vi "StartSession.vi"(8 "error in (no error)":errorcluster, 11 "TrialBasedExperiment in":refnum<class "MatlabExperiment.lvclass">) -> (0 "error out":errorcluster, 3 "TrialBasedExperiment out":refnum<class "MatlabExperiment.lvclass">)   [LabVIEW 2014, in "AcquisitionCoreObjects.lvlib" / "MatlabExperiment.lvclass"]
uses:
  MatlabExperiment.lvclass
  TrialBasedExperimentObject/TrialBasedExperiment.lvclass
  Matlab API/Matlab API.lvlib
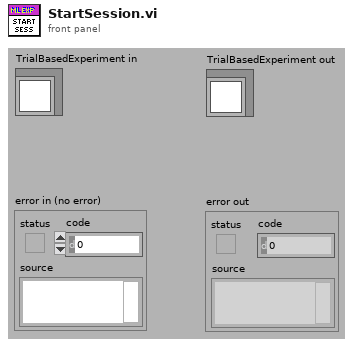
[diagram p1: front panel]
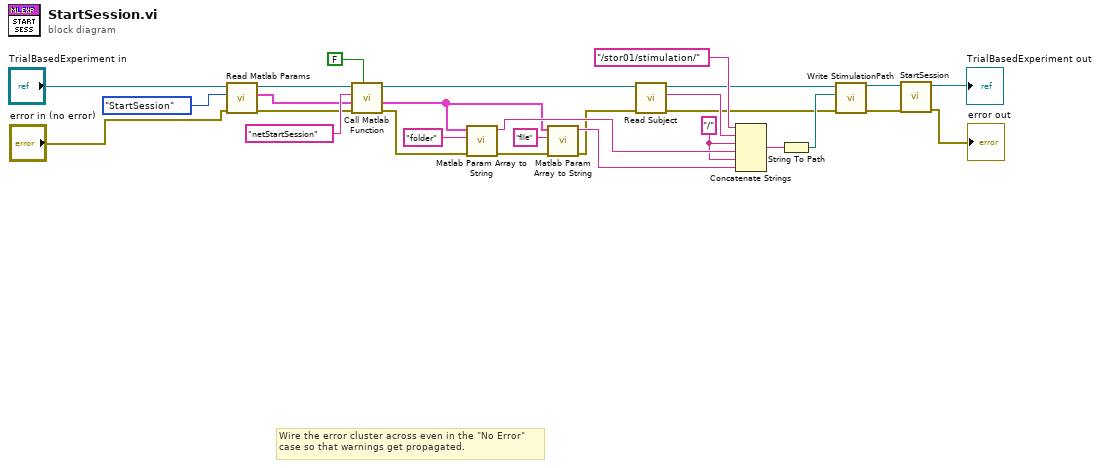
[diagram p0: block diagram]
diagram:
  w24 = "/" ("string")
  # "Wire the error cluster across even in the \"No Error\"\ncase so that warnings get propagated."
  n1 = call-dynamic "Read Matlab Params.vi"("error in (no error)"="error in (no error)", "Enum"=enum16{"StartSession", "StartTrial"}."StartSession", "TrialBasedExperiment in"="TrialBasedExperiment in") -> ("error out"=w15:errorcluster, "Matlab Param Array"=w17:cluster{"Name":string, "Data":variant}[], "TrialBasedExperiment out"=w7:refnum<class "MatlabExperiment.lvclass">)  [unwired: 6 in]
  n2 = call-dynamic "Call Matlab Function.vi"("Timestamp"=FALSE, "error in (no error)"=w15, "Matlab Param Array"=w17, "Function name"="netStartSession", "TrialBasedExperiment in"=w7) -> ("error out"=w14:errorcluster, "Return value struct"=w16:cluster{"Name":string, "Data":variant}[], "TrialBasedExperiment out"=w6:refnum<class "MatlabExperiment.lvclass">)  [unwired: 3 in, 1 out]
  n3 = call "Matlab Param Array to String.vi"("error in (no error)"=w14, "Name"="folder", "Matlab Param Array"=w16) -> ("error out"=w22:errorcluster, "data"=w26:string)  [unwired: 7 out]
  n4 = call "Matlab Param Array to String.vi"("error in (no error)"=w22, "Name"="file", "Matlab Param Array"=w16) -> ("error out"=w12:errorcluster, "data"=w25:string)  [unwired: 7 out]
  n5 = call-dynamic "Read Subject.vi"("error in (no error)"=w12, "TrialBasedExperiment in"=w6) -> ("error out"=w8:errorcluster, "Subject"=w13:string, "TrialBasedExperiment out"=w9:refnum<class "MatlabExperiment.lvclass">)  [unwired: 7 in]
  n6 = Concatenate Strings("/stor01/stimulation/" ("string"), w13, w24, w26, w24, w25) -> (w11:string)
  n7 = String To Path(string=w11) -> (path=w10:path)
  n8 = call-dynamic "Write StimulationPath.vi"("error in (no error)"=w8, "StimulationPath"=w10, "MatlabExperiment in"=w9) -> ("error out"=w4:errorcluster, "MatlabExperiment out"=w5:refnum<class "MatlabExperiment.lvclass">)  [unwired: 7 in]
  n9 = call-parent "StartSession.vi"("error in (no error)"=w4, "TrialBasedExperiment in"=w5) -> ("error out"=→"error out":errorcluster, "TrialBasedExperiment out"=→"TrialBasedExperiment out":refnum<class "MatlabExperiment.lvclass">)  [unwired: 8 in]
